vi "Hybrid Distance.vi"(9 "Camera Distance\nfrom Ground (in)":dbl, 10 "Normalized Rect":T2, 11 "Camera Type":T1) -> (2 "Distance Back (ft)":dbl, 3 "Distance Right (ft)":dbl)   [LabVIEW 2015]
uses:
  Camera Types.ctl
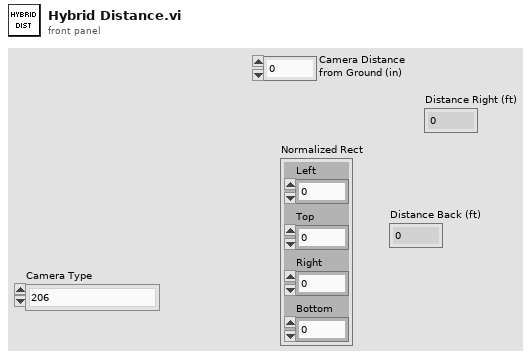
[diagram p1: front panel]
types:
  T1 = typedef "Camera Types.ctl" = enum16{"206", "1011", "1013", "MS HD3000 square", "MS HD3000 640x480"}
  T2 = cluster{"Left":dbl, "Top":dbl, "Right":dbl, "Bottom":dbl}
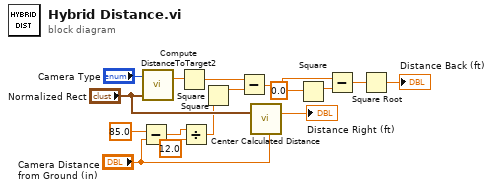
[diagram p0: block diagram]
diagram:
  n1 = Subtract(x=85.0, y="Camera Distance\nfrom Ground (in)") -> (x-y=w4:dbl)
  n2 = call "Compute DistanceToTarget2.vi"("Normalized Rect"="Normalized Rect", "Camera Type"="Camera Type") -> ("Distance (ft)"=w14:dbl)  [unwired: 9 in]
  n3 = Square(x=w14) -> (x^2=w13:dbl)
  n4 = Divide(x=w4, y=12.0) -> (x/y=w2:dbl)
  n5 = Square(x=w2) -> (x^2=w12:dbl)
  n6 = Subtract(x=w13, y=w12) -> (x-y=w11:dbl)
  n7 = call "Center Calculated Distance.vi"("Camera Distance\nfrom Ground (in)"="Camera Distance\nfrom Ground (in)", "Normalized Rect"="Normalized Rect") -> ("Distance Right (ft)"=→"Distance Right (ft)":dbl)  [unwired: 8 in, 1 out]
  n8 = Square(x=0.0) -> (x^2=w10:dbl)
  n9 = Subtract(x=w11, y=w10) -> (x-y=w8:dbl)
  n10 = Square Root(x=w8) -> (sqrt(x)=→"Distance Back (ft)":dbl)
